vi "StageControlTest.vi"() -> ()   [LabVIEW 2014]
doc: "This is to test each function of a stage. It would not be used in the main VI."
uses:
  C:/Users/light/Desktop/Peng/Raman/dll/Thorlabs.MotionControl.Controls.dll
  dll/Thorlabs.MotionControl.Controls.dll
  C:/Users/light/Desktop/Peng/Raman/dll/ThorLabs.MotionControl.KCube.DCServoCLI.dll
  dll/ThorLabs.MotionControl.KCube.DCServoCLI.dll
panel:
  in  "Item to test":enum16{"ReadPos", "ToPos"}(ring)
  in  "stop 2":bool
  in  "To Pos":dbl
  out "CurrentPosition":dbl
  out "error out":errorcluster
  in  "error in (no error)":errorcluster
  in  "stop":bool
  in  "KCubeDCServoControl":refnum<k24>(container)
  # "This is to test each function of a stage. It would not be used in the main VI."
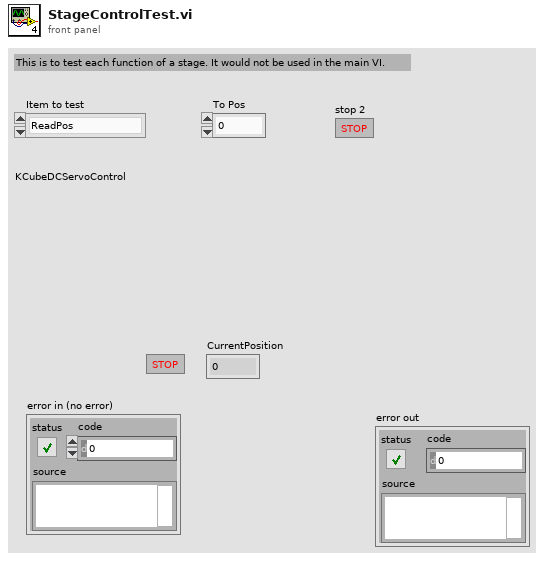
[diagram p1: front panel]
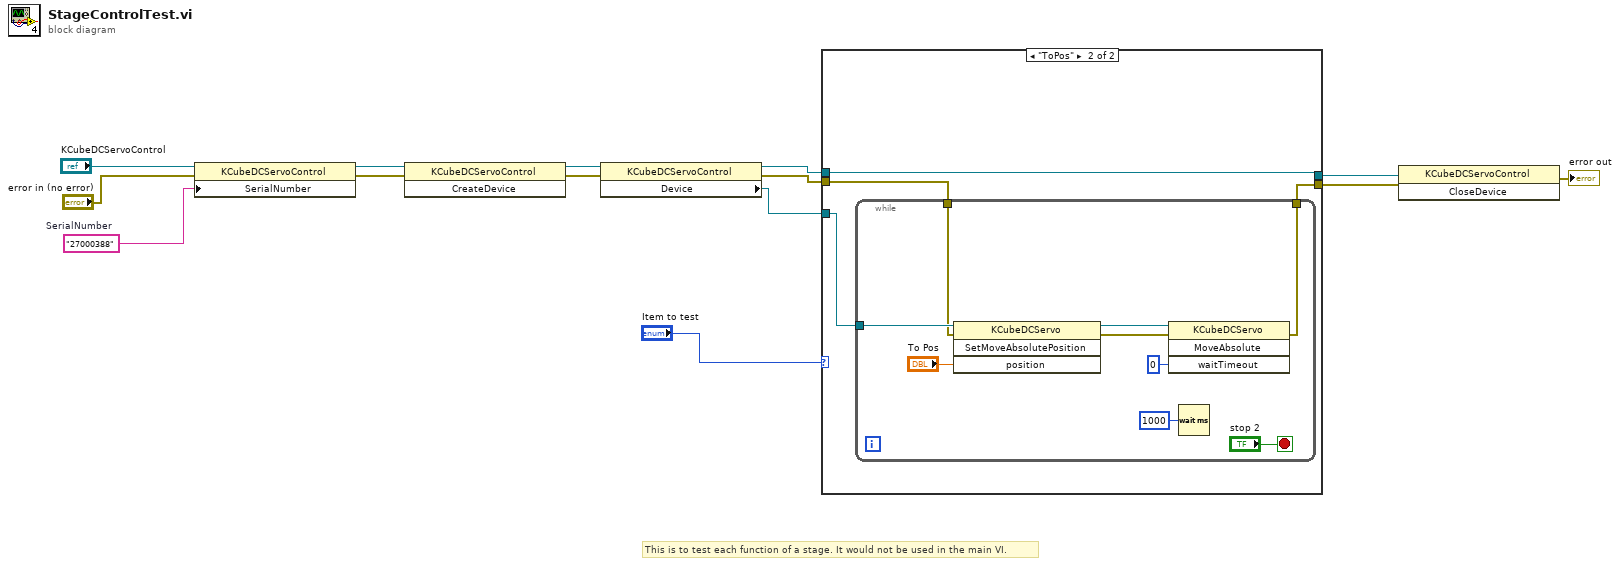
[diagram p0: block diagram]
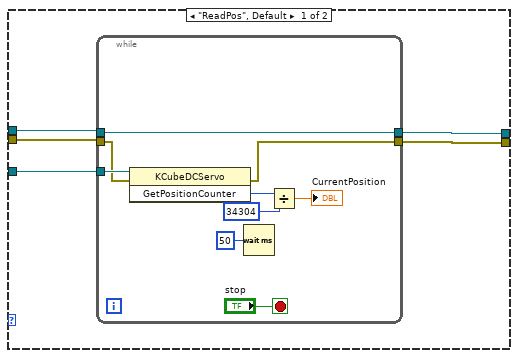
[diagram p2: hidden frame]
diagram:
  w13 = "27000388"  # SerialNumber
  # "This is to test each function of a stage. It would not be used in the main VI."
  n1 = property class="KCubeDCServoControl"(reference="KCubeDCServoControl", error in="error in (no error)", "SerialNumber"=w13) -> (reference out=w12:refnum<k24>, error out=w9:errorcluster)
  n2 = invoke class="KCubeDCServoControl" method="CreateDevice"(reference=w12, error in=w9) -> (reference out=w6:refnum<k24>, error out=w5:errorcluster)  [unwired: 1 in, 1 out]
  n3 = property class="KCubeDCServoControl"(reference=w6, error in=w5) -> (reference out=w4:refnum<k24>, error out=w3:errorcluster, "Device"=w2:refnum<k24>)
  n4 = case shown="\"ToPos\"" "Item to test" {
    tunnel: [w19 w31] -> w11
    tunnel: [w18 w29] -> w8
    tunnel: w4 -> [w17 w31]
    tunnel: w3 -> [w16 w30]
    tunnel: w2 -> [w15 w32]
    frame "ReadPos", Default {
      n5 = while {
        tunnel: [w27] -> w19
        tunnel: w17 -> [w27]
        tunnel: w16 -> [w21]
        tunnel: [w20] -> w18
        tunnel: w15 -> [w25]
        stop <- "stop" stop-if-true
        n6 = invoke class="KCubeDCServo" method="GetPositionCounter"(reference=w25, error in=w21) -> (error out=w20:errorcluster, "GetPositionCounter"=w24:i32)  [unwired: 1 in, 1 out]
        n7 = Wait (ms)(milliseconds to wait=u32 50) -> ()  [unwired: 1 out]
        n8 = Divide(x=w24, y=34304) -> (x/y=→"CurrentPosition":dbl)
      }
    }
    frame "ToPos" {
      n9 = while {
        tunnel: w32 -> [w35]
        tunnel: w30 -> [w34]
        tunnel: [w33] -> w29
        stop <- "stop 2" stop-if-true
        n10 = invoke class="KCubeDCServo" method="SetMoveAbsolutePosition"(reference=w35, error in=w34, "position"="To Pos") -> (reference out=w39:refnum<k24>, error out=w41:errorcluster)  [unwired: 1 in, 2 out]
        n11 = invoke class="KCubeDCServo" method="MoveAbsolute"(reference=w39, error in=w41, "waitTimeout"=0) -> (error out=w33:errorcluster)  [unwired: 1 in, 3 out]
        n12 = Wait (ms)(milliseconds to wait=u32 1000) -> ()  [unwired: 1 out]
      }
    }
  }
  n13 = invoke class="KCubeDCServoControl" method="CloseDevice"(reference=w11, error in=w8) -> (error out=→"error out":errorcluster)  [unwired: 1 in, 2 out]
